vi "Waveform Chart Update Type.vi"() -> ()   [LabVIEW 2020]
doc: "This VI illustrates the different kinds of charts and the data types that they can accept. Charts can accept a single point at a time or multiple points at a time. Also, charts can display multiple overlayed or stacked plots. To change between strip, scope, and sweep update modes, right click on the chart and select Advanced->Update Mode."
panel:
  out "Strip Chart":dbl(graph)
  out "Scope Chart":dbl(graph)
  out "Sweep Chart":dbl(graph)
  in  "Stop":bool
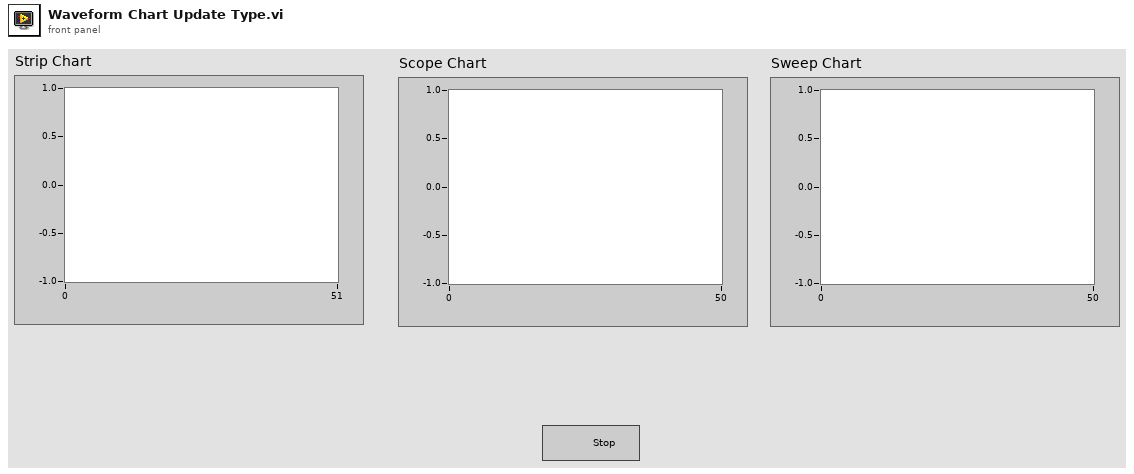
[diagram p1: front panel]
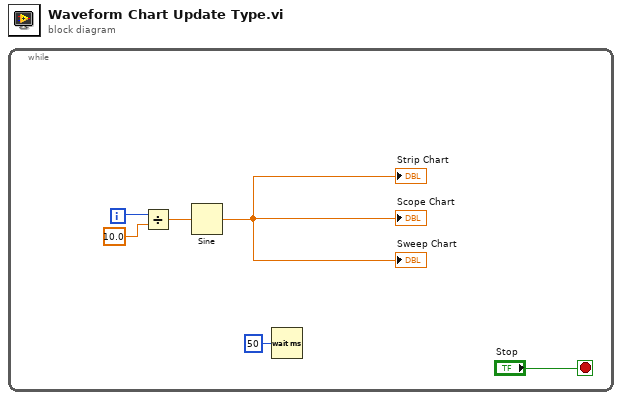
[diagram p0: block diagram]
diagram:
  n1 = while {
    i -> [w6]
    stop <- "Stop" stop-if-true
    # "Update Waveform Charts"
    n2 = Divide(x=w6, y=10.0) -> (x/y=w5:dbl)
    n3 = Sine(x=w5) -> (sin(x)=→"Sweep Chart" →"Scope Chart" →"Strip Chart":dbl)
    n4 = Wait (ms)(milliseconds to wait=u32 50 ("millisecond multiple")) -> ()  [unwired: 1 out]
  }
